vi "AMC e.bloxx Example - Write Digital Value.vi"() -> ()   [LabVIEW 2013]
doc: "<B>AMC - Analytik & Messtechnik GmbH Chemnitz</B>\n\nLabVIEW Drivers for e.bloxx series from Gantner Instruments\n\nThis example demonstrates the usage of the e.bloxx VIs. You must select your serial settings according to the e.bloxx configuration set via ICP software. Then choose your designated module by Module Address. This example displays a knight rider - style digital output pattern on 3 digital outputs. You can"
uses:
  AMC e.bloxx Write Value - Boolean.vi
panel:
  in  "Update Rate (ms)":u32=100
  out "error out":errorcluster
  in  "stop":bool
  in  "Module Address":i32=3
  in  "Parity":enum16{"None", "Odd", "Even", "Mark", "Space"}(ring)=enum."Even"
  in  "Baudrate":u32=115200
  in  "VISA Resource Name":refnum<visa-resource-name>="COM2"
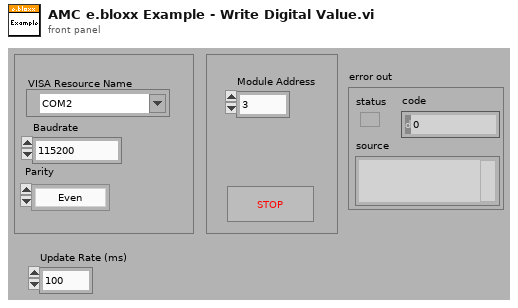
[diagram p1: front panel]
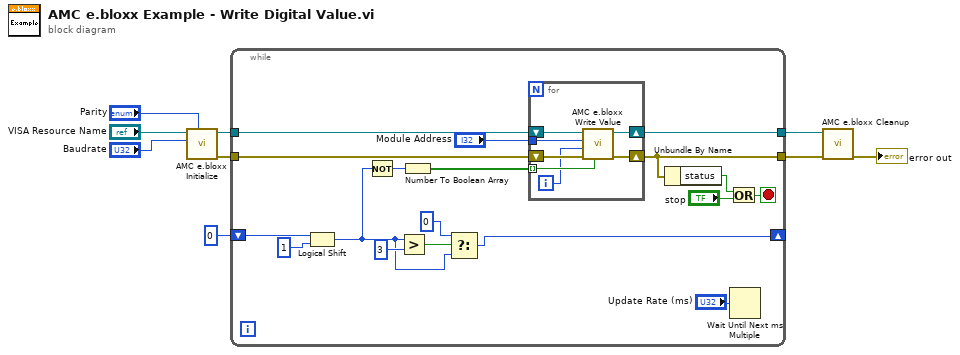
[diagram p0: block diagram]
diagram:
  n1 = call "AMC e.bloxx Initialize.vi"("parity (0:none)"="Parity", "baud rate (9600)"="Baudrate", "VISA resource name"="VISA Resource Name") -> ("error out"=w5:errorcluster, "VISA resource name out"=w6:refnum<visa-resource-name>)  [unwired: 7 in]
  n2 = while {
    tunnel: w6 -> [w27]
    tunnel: w5 -> [w26]
    tunnel: [w21] -> w4
    tunnel: [w20] -> w3
    shift-right: [w10] -> _
    shift-left: 0 -> [w18]
    stop <- w24 stop-if-true
    n3 = Logical Shift(y=w18, x=1) -> (x << y=w12:i32)
    n4 = Not(x=w12) -> (.not. x?=w16:i32)
    n5 = Greater?(x=w12, y=3) -> (0:w13:bool)
    n6 = Number To Boolean Array(number=w16) -> (Boolean array=w15:bool[])
    n7 = Select(t=0, s=w13, f=w12) -> (s? t:f=w10:i32)
    n8 = for {
      tunnel: "Module Address" -> [w32]
      shift-right: [w31] -> w21
      shift-left: w27 -> [w34]
      shift-right: [w30] -> w20
      shift-left: w26 -> [w33]
      tunnel: w15 -> [w29] mode=indexing
      i -> [w28]
      n9 = call-poly "AMC e.bloxx Write Value.vi"("Value"=w29, "error in (no error)"=w33, "Channel"=w28, "Module Address"=w32, "VISA Resource Name"=w34) -> ("error out"=w30:errorcluster, "VISA Resource Name out"=w31:refnum<visa-resource-name>)  [unwired: 5 in]
    }
    n10 = Unbundle By Name(w20) -> ("status"=w22:bool)
    n11 = Or(x=w22, y="stop") -> (x .or. y?=w24:bool)
    n12 = Wait Until Next ms Multiple(millisecond multiple="Update Rate (ms)") -> ()  [unwired: 1 out]
  }
  n13 = call "AMC e.bloxx Cleanup.vi"("error in (no error)"=w3, "VISA resource name"=w4) -> ("error out"=→"error out":errorcluster)  [unwired: 9 in]
